vi "Show User Interface.vi"(8 "error in (no error)":errorcluster, 9 "Process VI Refnums":refnum<vi>[](array[refnum]), 10 "Show UI":bool, 11 "SMO.UI":refnum<class "SMO.UI.Template.lvclass">) -> (0 "error out":errorcluster, 3 "SMO.UI out":refnum<class "SMO.UI.Template.lvclass">)   [LabVIEW 2013, in "SMO.UI.Template.lvclass"]
uses:
  SMO.UI.Template.lvclass
  SMO.UI/SMO.UI.lvclass
  SMO/SMO.lvclass
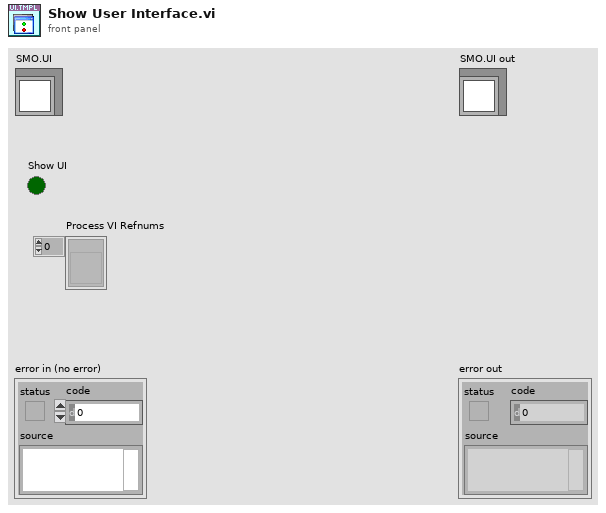
[diagram p1: front panel]
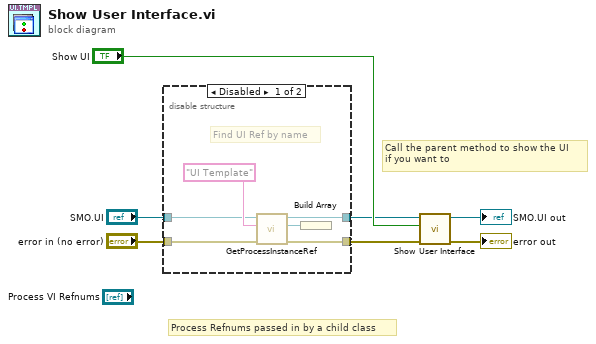
[diagram p0: block diagram]
diagram:
  # "Process Refnums passed in by a child class"
  # "Call the parent method to show the UI\nif you want to"
  n1 = disable-structure shown="Disabled" {
    disable-tunnel: "SMO.UI" -> [w11 w14]
    disable-tunnel: "error in (no error)" -> [w9 w13]
    disable-tunnel: [w9 w13] -> w2
    disable-tunnel: [w8 w14] -> w1
    frame Disabled {
      # "Find UI Ref by name"
      n2 = call "GetProcessInstanceRef.vi"("Process Name"="UI Template", "SMO"=w11) -> ("Process VI Refnum"=w10:refnum<vi>, "SMO out"=w8:refnum<class "SMO.UI.Template.lvclass">)  [unwired: 7 in, 1 out]
      n3 = Build Array(w10) -> ()  [unwired: 1 out]
    }
    frame Enabled {
      # "The SMO.UI will open\nthe UI of the lowest child"
    }
  }
  n4 = call-parent "Show User Interface.vi"("error in (no error)"=w2, "Show UI"="Show UI", "SMO.UI"=w1) -> ("error out"=→"error out":errorcluster, "SMO.UI out"=→"SMO.UI out":refnum<class "SMO.UI.Template.lvclass">)  [unwired: 7 in]
